vi "confirmation_user.vi"(6 "VI Description":string, 7 "Indicator/Control":bool[](array[boolean]), 8 "error in (no error)":errorcluster, 9 "Tip Strips":string[](array[string]), 10 "Descriptions":string[](array[string]), 11 "Control Labels":string[](array[string])) -> (0 "error out":errorcluster, 1 "Update VI Desc":bool, 3 "Selected Controls":i32[](array[numeric]), 5 "Update":bool)   [LabVIEW 2020, in "lv_documentation.lvlib"]
uses:
  lv_documentation.lvlib
panel:
  in  "Cancel":bool
  in  "Update":bool
  in  "Select VI Desc":bool
  out "VI Description":string caption="Update VI Description"
  out "Indicators List":i32(listbox)
  out "Controls List":i32(listbox)
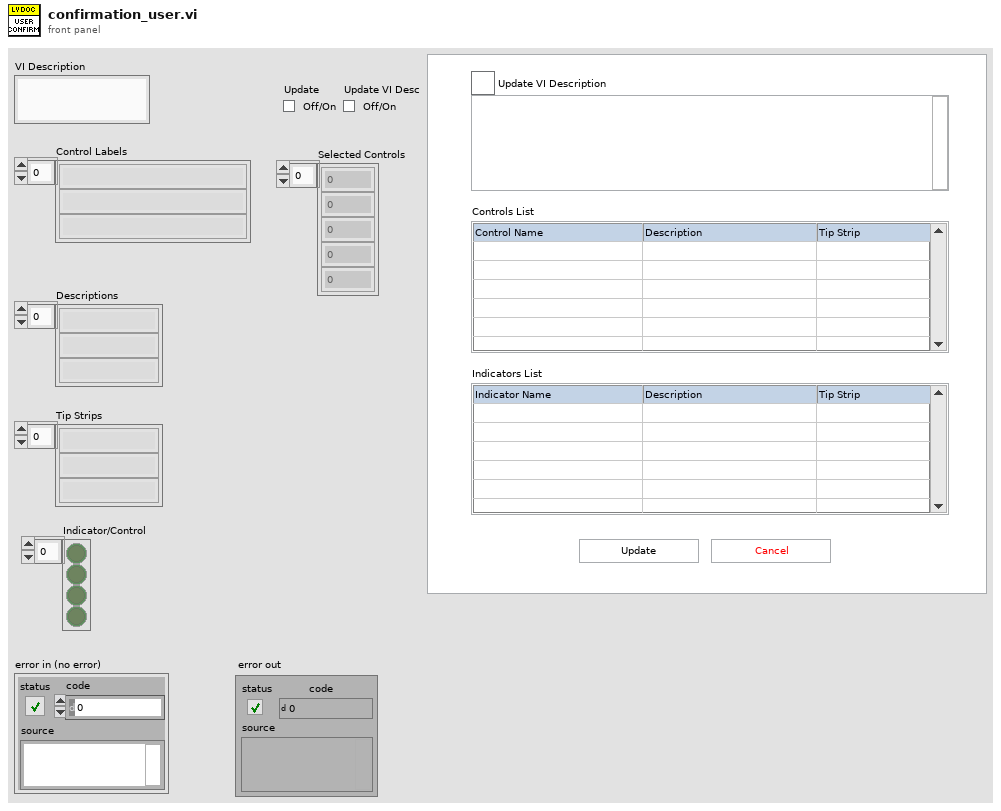
[diagram p1: front panel]
types:
  T1 = typedef "LVPoint32TypeDef.ctl" = cluster{"Horizontal":i32, "Vertical":i32}
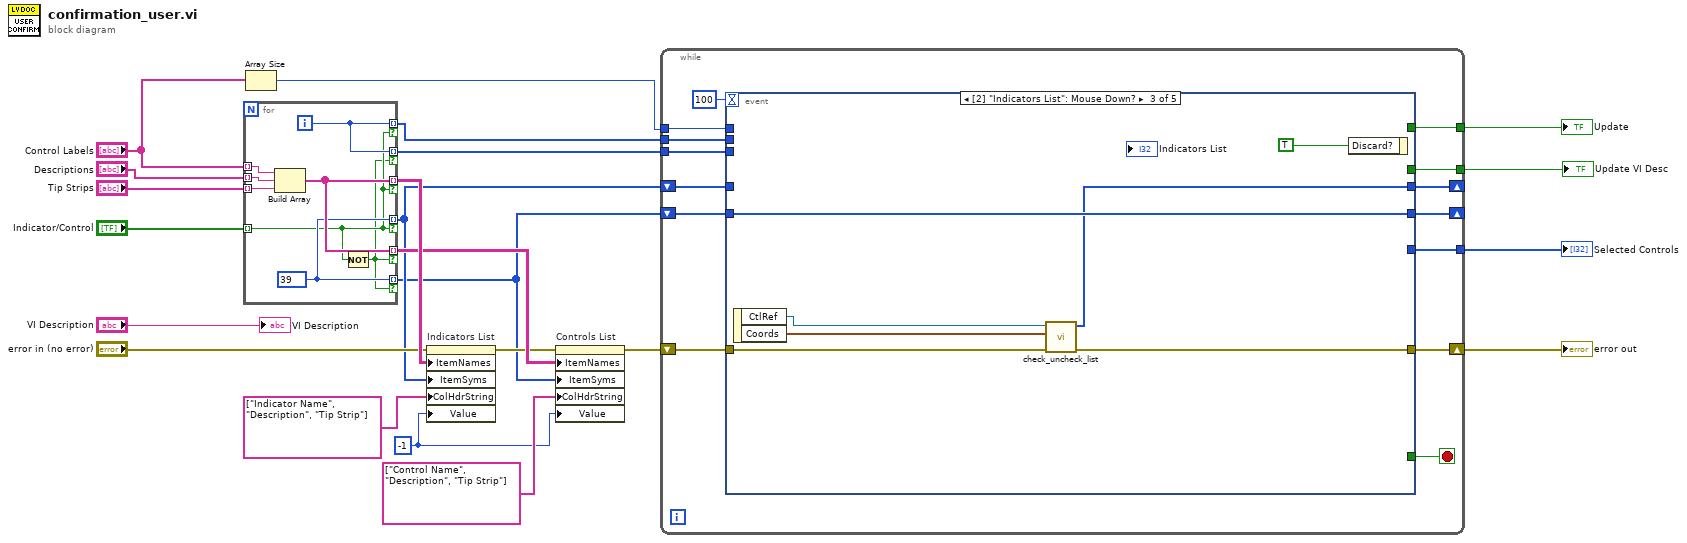
[diagram p0: block diagram]
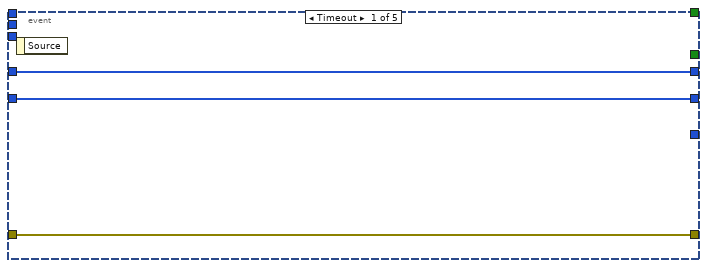
[diagram p2: hidden frame]
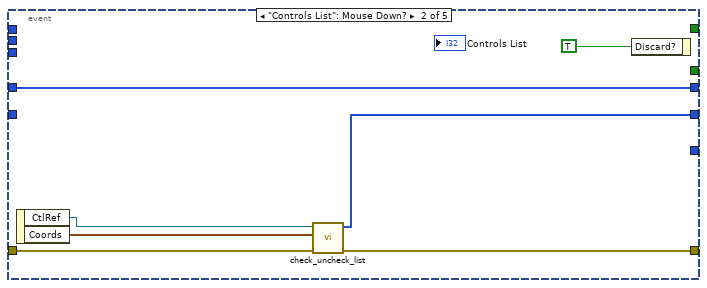
[diagram p3: hidden frame]
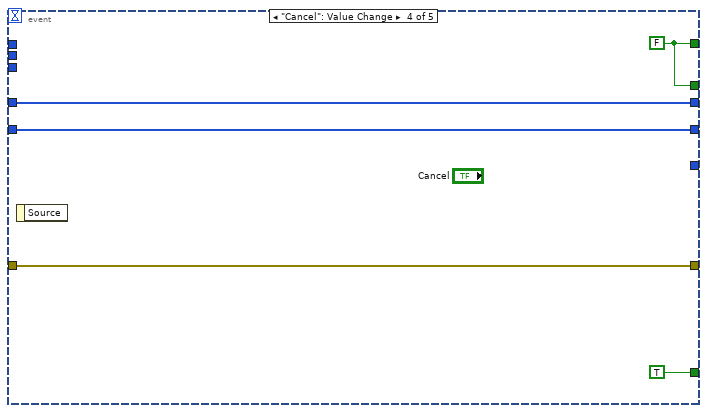
[diagram p4: hidden frame]
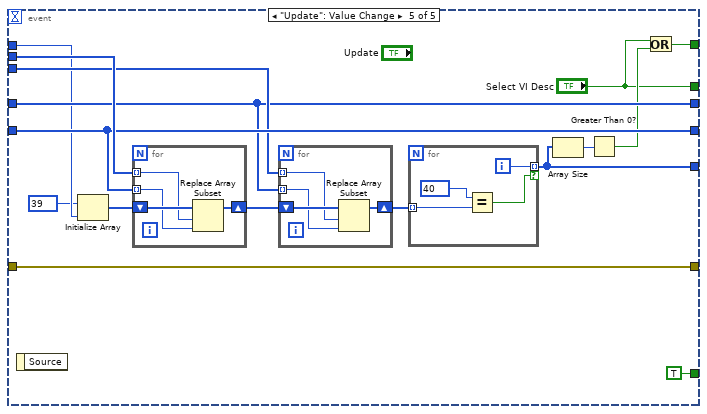
[diagram p5: hidden frame]
diagram:
  w12 = -1 ("Indicators List")
  n1 = for {
    tunnel: "Control Labels" -> [w30] mode=indexing
    tunnel: "Descriptions" -> [w29] mode=indexing
    tunnel: "Tip Strips" -> [w28] mode=indexing
    tunnel: [w27] -> w20 mode=indexing if=w24
    tunnel: [w26] -> w9 mode=indexing if=w24
    tunnel: "Indicator/Control" -> [w24] mode=indexing
    tunnel: [w27] -> w18 mode=indexing if=w23
    tunnel: [w26] -> w8 mode=indexing if=w23
    tunnel: [w25] -> w7 mode=indexing if=w24
    tunnel: [w25] -> w6 mode=indexing if=w23
    i -> [w25]
    w26 = 39
    n2 = Build Array(w30, w29, w28) -> (w27:string[])
    n3 = Not(x=w24) -> (.not. x?=w23:bool)
  }
  n4 = Array Size(array="Control Labels") -> (size(s)=w4:i32)
  n5 = property on="Indicators List" class="MCListbox (strict)"(error in="error in (no error)", "ItemNames"=w20, "ItemSyms"=w9, "ColHdrString"=string[] ["Indicator Name", "Description", "Tip Strip"] ("Row Header Strings[]"), "Value"=w12) -> (error out=w17:errorcluster)  [unwired: 1 in, 1 out]
  n6 = property on="Controls List" class="MCListbox (strict)"(error in=w17, "ItemNames"=w18, "ItemSyms"=w8, "ColHdrString"=string[] ["Control Name", "Description", "Tip Strip"] ("Row Header Strings[]"), "Value"=w12) -> (error out=w11:errorcluster)  [unwired: 1 in, 1 out]
  n7 = while {
    shift-right: [w42] -> w10
    shift-left: w11 -> [w43]
    shift-right: [w38] -> _
    shift-left: w8 -> [w40]
    shift-right: [w39] -> _
    shift-left: w9 -> [w41]
    tunnel: [w37] -> w2
    tunnel: w7 -> [w35]
    tunnel: w6 -> [w34]
    tunnel: w4 -> [w33]
    tunnel: [w32] -> w3
    tunnel: [w31] -> w1
    stop <- w36 stop-if-true
    n8 = event shown="[2] \"Indicators List\": Mouse Down?" {
      selector: _ -> [_ _ _ _ _]
      dyn-events: _ -> [_ _ _ _ _]
      timeout: 100 -> [_ _ _ _ _]
      tunnel: w43 -> [w47 w50 w61 w66 w82]
      tunnel: [w47 w49 w56 w66 w82] -> w42
      tunnel: w41 -> [w46 w54 _ w65 w76]
      tunnel: w40 -> [w45 _ w58 w64 w79]
      tunnel: [w46 w54 w55 w65 w76] -> w39
      tunnel: [w45 w48 w58 w64 w79] -> w38
      tunnel: [_ _ _ w62 w69] -> w37
      tunnel: [_ _ _ TRUE TRUE] -> w36
      tunnel: w35 -> [_ _ _ _ w80]
      tunnel: w34 -> [_ _ _ _ w77]
      tunnel: w33 -> [_ _ _ _ w68]
      tunnel: [_ _ _ _ w73] -> w32
      tunnel: [_ _ _ w62 "Select VI Desc"] -> w31
      event Timeout {
        n9 = event-data() -> ()  [unwired: 1 in, 1 out]
      }
      event "Controls List": Mouse Down? {
        n10 = event-data() -> ("CtlRef"=w52:refnum<vi>, "Coords"=w51:T1)  [unwired: 1 in]
        n11 = call "check_uncheck_list.vi"("error in (no error)"=w50, "Coords"=w51, "MulticolumnListbox in"=w52) -> ("error out"=w49:errorcluster, "ItemSyms"=w48:i32[])  [unwired: 7 in]
        n12 = event-data("Discard?"=TRUE) -> ()  [unwired: 1 in, 1 out]
      }
      event "Indicators List": Mouse Down? {
        n13 = event-data() -> ("CtlRef"=w60:refnum<vi>, "Coords"=w59:T1)  [unwired: 1 in]
        n14 = call "check_uncheck_list.vi"("error in (no error)"=w61, "Coords"=w59, "MulticolumnListbox in"=w60) -> ("error out"=w56:errorcluster, "ItemSyms"=w55:i32[])  [unwired: 7 in]
        n15 = event-data("Discard?"=TRUE) -> ()  [unwired: 1 in, 1 out]
      }
      event "Cancel": Value Change {
        w62 = FALSE
        n16 = event-data() -> ()  [unwired: 1 in, 1 out]
      }
      event "Update": Value Change {
        n17 = event-data() -> ()  [unwired: 1 in, 1 out]
        n18 = Initialize Array(39, w68) -> (w78:i32[])
        n19 = for {
          tunnel: w80 -> [w93] mode=indexing
          tunnel: w79 -> [w92] mode=indexing
          shift-right: [w91] -> w75
          shift-left: w78 -> [w94]
          n20 = Replace Array Subset(array=w94, new element=w92, index=w93) -> (w91:i32[])
        }
        n21 = for {
          tunnel: w77 -> [w89] mode=indexing
          tunnel: w76 -> [w88] mode=indexing
          shift-right: [w87] -> w74
          shift-left: w75 -> [w90]
          n22 = Replace Array Subset(array=w90, new element=w88, index=w89) -> (w87:i32[])
        }
        n23 = for {
          tunnel: w74 -> [w86] mode=indexing
          tunnel: [w84] -> w73 mode=indexing if=w83
          i -> [w84]
          n24 = Equal?(x=40, y=w86) -> (x = y?=w83:bool)
        }
        n25 = Array Size(array=w73) -> (size(s)=w72:i32)
        n26 = Greater Than 0?(x=w72) -> (x > 0?=w71:bool)
        n27 = Or(x="Select VI Desc", y=w71) -> (x .or. y?=w69:bool)
      }
    }
  }
  "error out" <- w10
  "Selected Controls" <- w3
  "Update" <- w2
  "Update VI Desc" <- w1
  "VI Description" <- "VI Description"
